vi "Prep Backsave Directory.vi"(8 "Error In":errorcluster, 11 "Revert Config":T1={"Revert Paths"={"Archive Path"=path "D:/workspace/revert/todo/todo.zip", "Unzip Directory"=path "D:/workspace/revert/unzip", "Backsave Directory"=path "D:/workspace/revert/backsave", "Output Archive"=path "D:/workspace/revert/backsave", "Backsave Common Directory"=path "D:/workspace/revert/backsave"}, "LabVIEW Files"={"Projects"=[], "Libraries"=[], "Classes"=[], "XControls"=[], "VIs and Controls"=[], "Non LV Files"=[]}, "LabVIEW Version"=enum."8.0"}) -> (0 "Error Out":errorcluster, 3 "Revert Config":T1={"Revert Paths"={"Archive Path"=path "D:/workspace/revert/todo/todo.zip", "Unzip Directory"=path "D:/workspace/revert/unzip", "Backsave Directory"=path "D:/workspace/revert/backsave", "Output Archive"=path "D:/workspace/revert/backsave", "Backsave Common Directory"=path "D:/workspace/revert/backsave"}, "LabVIEW Files"={"Projects"=[], "Libraries"=[], "Classes"=[], "XControls"=[], "VIs and Controls"=[], "Non LV Files"=[]}, "LabVIEW Version"=enum."8.0"})   [LabVIEW 2013, in "LVH-Revert.lvlib"]
uses:
  LVH-Revert.lvlib
  Type Defs/Revert Config.ctl
  Type Defs/Paths.ctl
  Type Defs/LabVIEW Files.ctl
  <vilib>/LabVIEW Hacker/LVH-Toolbox/Common/Private/Type Defs/LabVIEW Version.ctl
  <vilib>/LabVIEW Hacker/LVH-Toolbox/Common/LVH-Common.lvlib
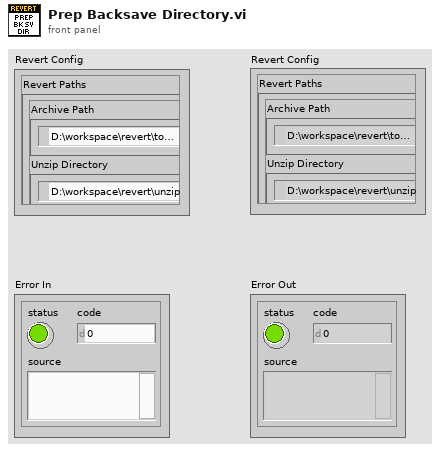
[diagram p1: front panel]
types:
  T1 = typedef "LVH-Revert.lvlib/Revert Config.ctl" = cluster{"Revert Paths":T2, "LabVIEW Files":T3, "LabVIEW Version":T4}
  T2 = typedef "LVH-Revert.lvlib/Paths.ctl" = cluster{"Archive Path":path, "Unzip Directory":path, "Backsave Directory":path, "Output Archive":path, "Backsave Common Directory":path}
  T3 = typedef "LVH-Revert.lvlib/LabVIEW Files.ctl" = cluster{"Projects":path[], "Libraries":path[], "Classes":path[], "XControls":path[], "VIs and Controls":path[], "Non LV Files":path[]}
  T4 = typedef "LVH-Toolbox.lvlib/LVH-Common.lvlib/LabVIEW Version.ctl" = enum16{"8.0", "8.2", "8.6", "9.0", "10.0", "11.0", "12.0", "13.0"}
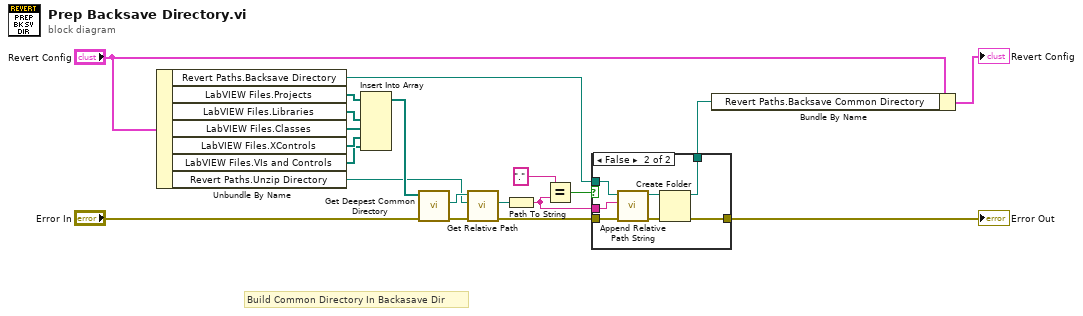
[diagram p0: block diagram]
diagram:
  # "Build Common Directory In Backasave Dir"
  n1 = Unbundle By Name("Revert Config") -> ("Revert Paths.Backsave Directory"=w9:path, "LabVIEW Files.Projects"=w20:path[], "LabVIEW Files.Libraries"=w19:path[], "LabVIEW Files.Classes"=w18:path[], "LabVIEW Files.XControls"=w17:path[], "LabVIEW Files.VIs and Controls"=w16:path[], "Revert Paths.Unzip Directory"=w11:path)
  n2 = Insert Into Array(array=w20, new element #1=w19, new element #2=w18, new element #3=w17, new element #4=w16) -> (w15:path[])  [unwired: 1 in]
  n3 = call <vilib>:"Get Deepest Common Directory.vi"("Error In"="Error In", "File Paths"=w15) -> ("Error Out"=w12:errorcluster, "Deepest Common Path"=w13:path)  [unwired: 7 in, 1 out]
  n4 = call <vilib>:"Get Relative Path.vi"("Error In"=w12, "Relative Path Root"=w11, "File / Folder"=w13) -> ("Error Out"=w8:errorcluster, "Relative Path"=w10:path)  [unwired: 6 in, 1 out]
  n5 = Path To String(path=w10) -> (string=w1:string)
  n6 = Equal?(x=".", y=w1) -> (x = y?=w2:bool)
  n7 = case shown="False" w2 {
    tunnel: w9 -> [w21 w29]
    tunnel: w8 -> [w22 w28]
    tunnel: [w22 w25] -> w7
    tunnel: [w21 w24] -> w4
    tunnel: w1 -> [_ w23]
    frame True {
    }
    frame False {
      n8 = call <vilib>:"Append Relative Path String.vi"("Error In"=w28, "Relative Path"=w23, "Base Path"=w29) -> ("Error Out"=w27:errorcluster, "Absolute Path"=w26:path)  [unwired: 7 in]
      n9 = Create Folder(path (use dialog)=w26, error in=w27) -> (created path=w24:path, error out=w25:errorcluster)  [unwired: 1 in, 1 out]
    }
  }
  "Error Out" <- w7
  n10 = Bundle By Name(cluster="Revert Config", "Revert Paths.Backsave Common Directory"=w4) -> (→"Revert Config":T1)
